vi "Read_Double_Vals.vi"() -> ()   [LabVIEW 2020]
uses:
  <vilib>/Utility/file.llb/Read Delimited Spreadsheet (DBL).vi
panel:
  out "first row":dbl[](array[numeric]) format="%#_4f"
  out "error out":errorcluster
  out "Read values":dbl[][](array[numeric]) format="%#_4f"
  out "Path":path
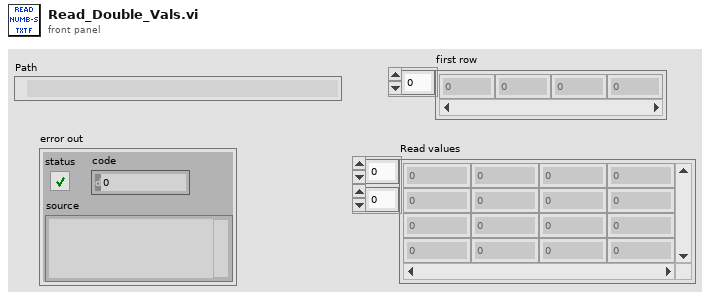
[diagram p1: front panel]
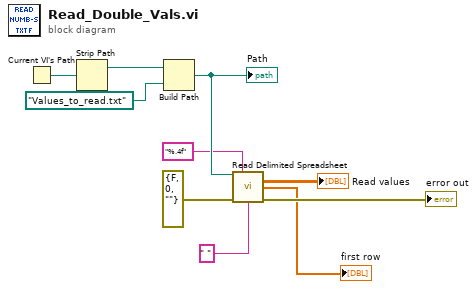
[diagram p0: block diagram]
diagram:
  n1 = Current VI's Path() -> (path=w10:path)
  n2 = Strip Path(path=w10) -> (stripped path=w9:path)  [unwired: 1 out]
  n3 = Build Path(base path=w9, name or relative path=path "Values_to_read.txt") -> (appended path=w7:path)
  "Path" <- w7
  n4 = call-poly <vilib>:"Read Delimited Spreadsheet.vi"("file path (dialog if empty)"=w7, "format (%.3f)"="%.4f", "error in (no error)"=errorcluster {"status"=FALSE, "code"=0, "source"=""}, "delimiter (\\t)"=" " ("delimiter (\\t)")) -> ("all rows"=→"Read values":dbl[][], "first row"=→"first row":dbl[], "error out"=→"error out":errorcluster)  [unwired: 6 in, 3 out]
